vi "Init.vi"(8 "error in (no error)":errorcluster, 11 "DisplaySize":T1) -> (0 "error out":errorcluster, 3 "Feeder out":refnum<class "Feeder.lvclass">)   [LabVIEW 2018, in "Feeder.lvclass"]
uses:
  Feeder.lvclass
  Typedefs/DisplaySize.ctl
  Feeder.lvclass/Feeder.ctl
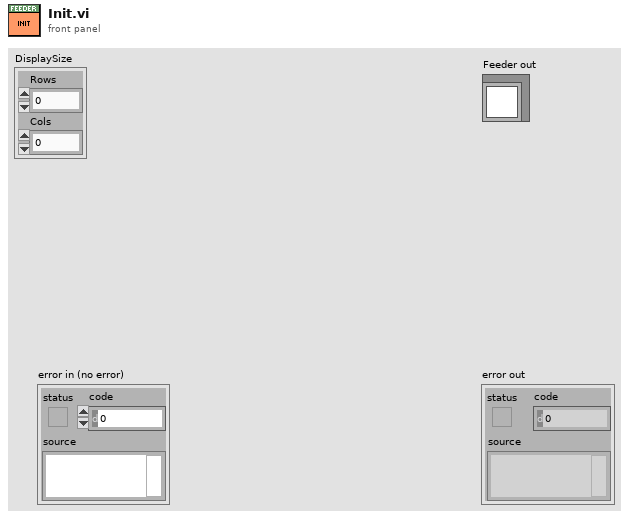
[diagram p1: front panel]
types:
  T1 = typedef "DisplaySize.ctl" = cluster{"Rows":i32, "Cols":i32}
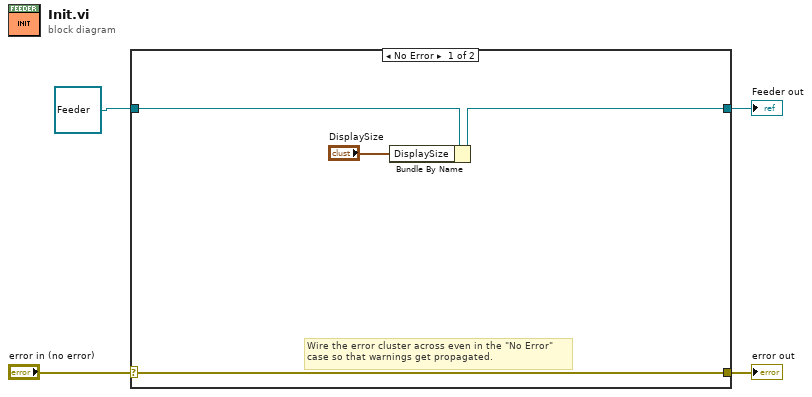
[diagram p0: block diagram]
diagram:
  n1 = case shown="No Error" "error in (no error)" {
    selector: "error in (no error)" -> [w7 w10]
    tunnel: [w7 w10] -> w3
    tunnel: [w6 w9] -> w1
    tunnel: refnum<class "Feeder.lvclass"> refnum ("Feeder in") -> [w8 w9]
    frame No Error {
      # "Wire the error cluster across even in the \"No Error\"\ncase so that warnings get propagated."
      n2 = Bundle By Name(cluster=w8, "DisplaySize"="DisplaySize") -> (w6:refnum<class "Feeder.lvclass">)
    }
    frame Error {
    }
  }
  "error out" <- w3
  "Feeder out" <- w1
